vi "WF_Load_single_file.vi"(9 "Limit for Stop file#":dbl, 10 "Enable limit = True":bool, 11 "WF_FILE_IN":path) -> (0 "Stop":bool, 1 "dt":dbl, 2 "Record#":i32, 3 "Waveform":waveform(dbl), 4 "File_duration(s)":dbl)   [LabVIEW 2017]
uses:
  <vilib>/Waveform/WDTFileIO.llb/Read Waveform from File.vi
  <vilib>/Waveform/WDTOps.llb/WDT Append Waveforms DBL.vi
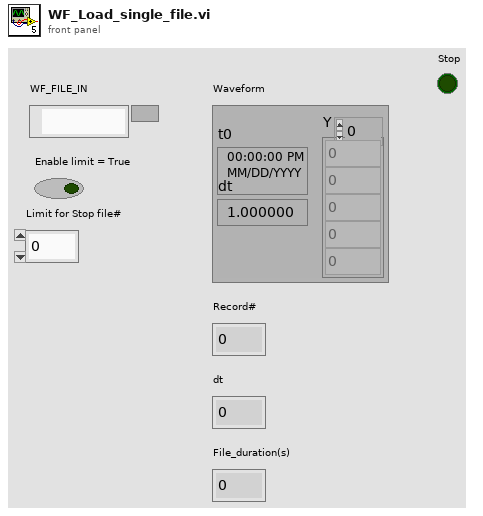
[diagram p1: front panel]
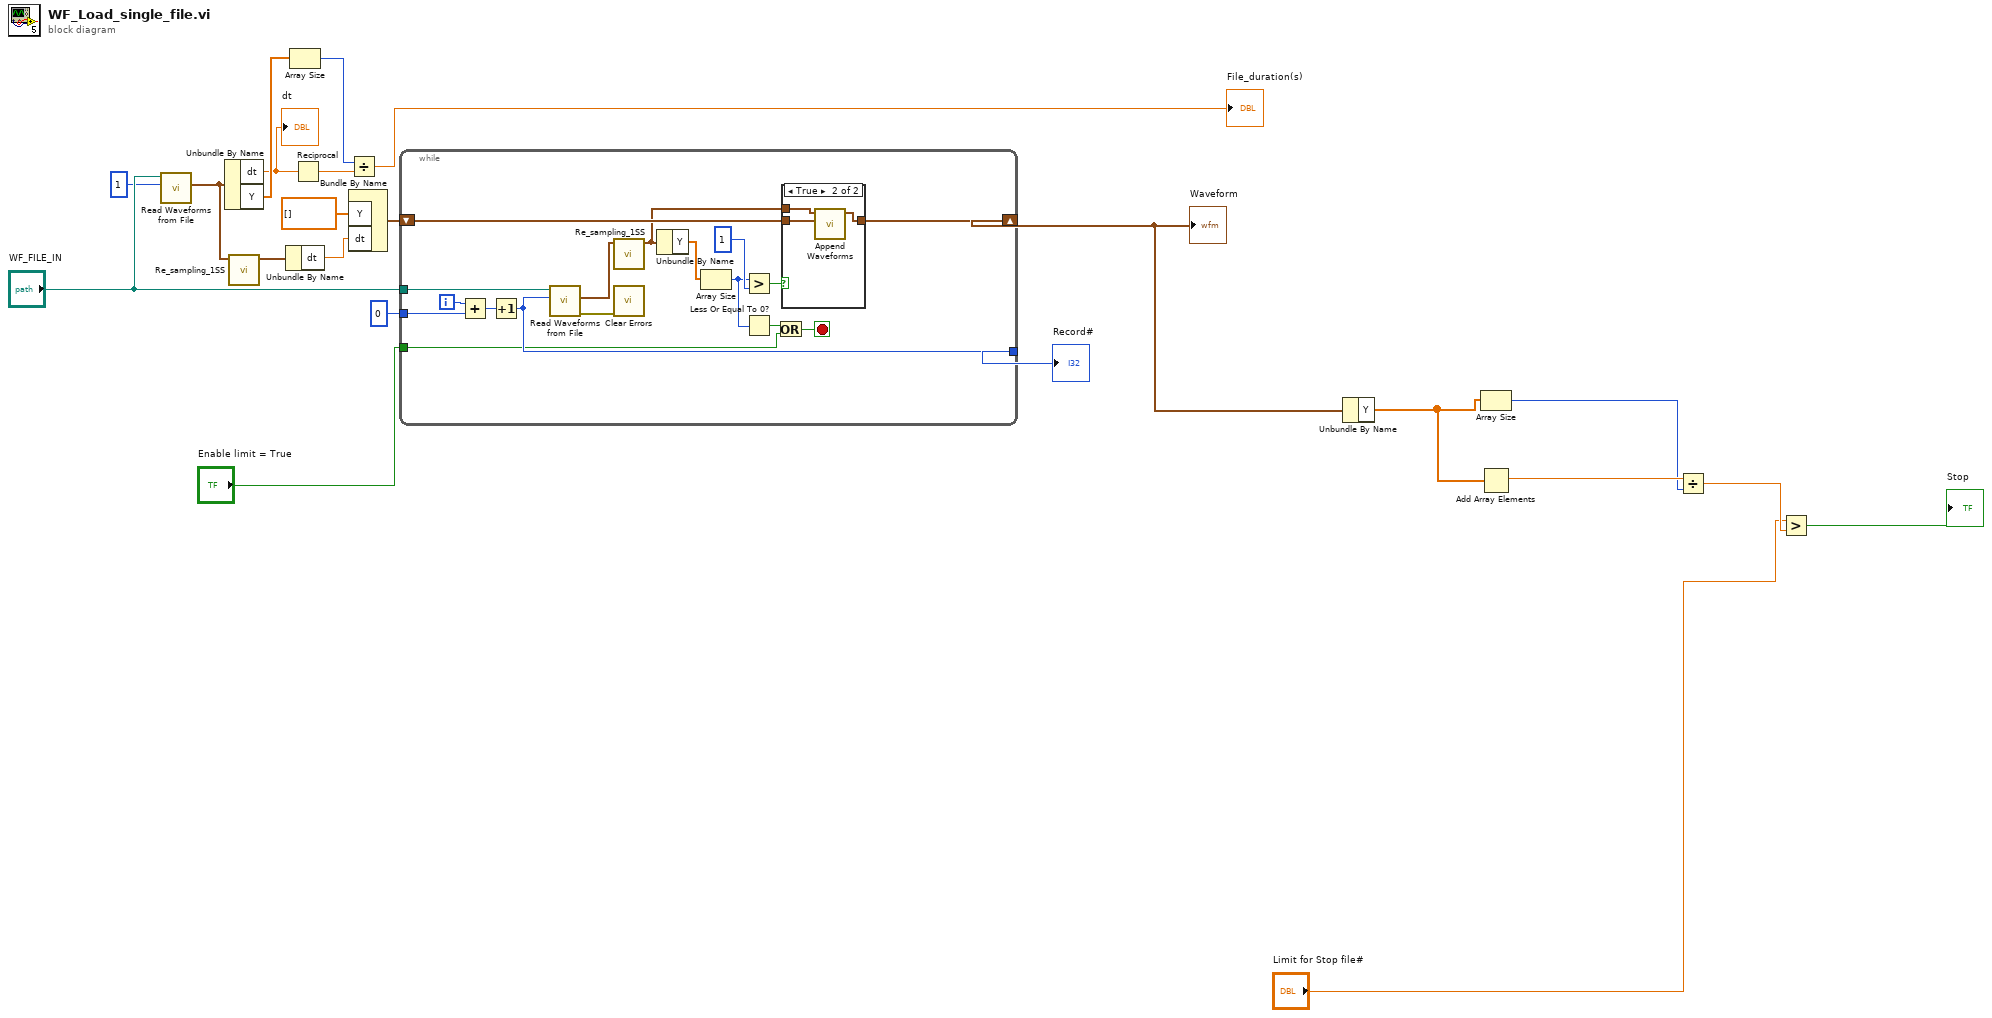
[diagram p0: block diagram]
diagram:
  n1 = call-poly <vilib>:"Read Waveforms from File.vi"("offset (records:0)"=1, "file path (dialog if empty)"="WF_FILE_IN") -> ("first waveform in record"=w16:waveform(dbl))  [unwired: 4 in, 3 out]
  n2 = Unbundle By Name(w16) -> ("dt"=w17:dbl, "Y"=w18:dbl[])
  "dt" <- w17
  n3 = call "Re_sampling_1SS.vi"("Waveform_main"=w16) -> ("Waveform"=w14:waveform(dbl))  [unwired: 10 in]
  n4 = Unbundle By Name(w14) -> ("dt"=w10:dbl)
  n5 = Array Size(array=w18) -> (size(s)=w19:i32)
  n6 = Reciprocal(x=w17) -> (1/x=w20:dbl)
  n7 = Divide(x=w19, y=w20) -> (x/y=→"File_duration(s)":dbl)
  n8 = Bundle By Name("Y"=dbl[] [], "dt"=w10) -> (w11:waveform(dbl))  [unwired: 1 in]
  n9 = while {
    shift-right: [w39] -> w7
    shift-left: w11 -> [w35]
    tunnel: "WF_FILE_IN" -> [w38]
    tunnel: "Enable limit = True" -> [w24]
    tunnel: [w28] -> w15
    tunnel: 0 ("y") -> [w23]
    i -> [w26]
    stop <- w34 stop-if-true
    n10 = Add(x=w26, y=w23) -> (x+y=w25:i32)
    n11 = Increment(x=w25) -> (x+1=w28:i32)
    n12 = call-poly <vilib>:"Read Waveforms from File.vi"("offset (records:0)"=w28, "file path (dialog if empty)"=w38) -> ("error out"=w36:errorcluster, "first waveform in record"=w27:waveform(dbl))  [unwired: 4 in, 2 out]
    n13 = call "Re_sampling_1SS.vi"("Waveform_main"=w27) -> ("Waveform"=w33:waveform(dbl))  [unwired: 10 in]
    n14 = call <vilib>:"Clear Errors.vi"("error in (no error)"=w36) -> ()  [unwired: 5 in, 2 out]
    n15 = Unbundle By Name(w33) -> ("Y"=w37:dbl[])
    n16 = Array Size(array=w37) -> (size(s)=w30:i32)
    n17 = Greater?(x=w30, y=1) -> (0:w31:bool)
    n18 = Less Or Equal To 0?(x=w30) -> (x <= 0?=w29:bool)
    n19 = Or(x=w29, y=w24) -> (x .or. y?=w34:bool)
    n20 = case shown="True" w31 {
      tunnel: [w40 w43] -> w39
      tunnel: w33 -> [_ w41]
      tunnel: w35 -> [w40 w42]
      frame False {
      }
      frame True {
        n21 = call-poly <vilib>:"Append Waveforms.vi"("waveform B"=w42, "waveform A"=w41) -> ("waveform out"=w43:waveform(dbl))  [unwired: 8 in, 1 out]
      }
    }
  }
  "Record#" <- w15
  "Waveform" <- w7
  n22 = Unbundle By Name(w7) -> ("Y"=w6:dbl[])
  n23 = Array Size(array=w6) -> (size(s)=w4:i32)
  n24 = Add Array Elements(numeric array=w6) -> (sum=w5:dbl)
  n25 = Divide(x=w5, y=w4) -> (x/y=w2:dbl)
  n26 = Greater?(x="Limit for Stop file#", y=w2) -> (0:→"Stop":bool)
